vi "Check Refnum Class.vi"(8 "error in (no error)":errorcluster, 11 "Ring Field in":refnum<class "Ring Field.lvclass">) -> (0 "error out":errorcluster, 3 "Ring Field out":refnum<class "Ring Field.lvclass">)   [LabVIEW 2020, in "Basic Fields.lvlib" / "Ring Field.lvclass"]
uses:
  Ring Field.lvclass
  C:/Users/User/Desktop/Raman Program/Database OOP/source/Field/Field Class/Field.lvclass
  Field/Field Class/Field.lvclass/Field.ctl
  Field/Field Class/Field.lvclass
panel:
  # "For override: make sure that the wired control refnum class matches the field child class"
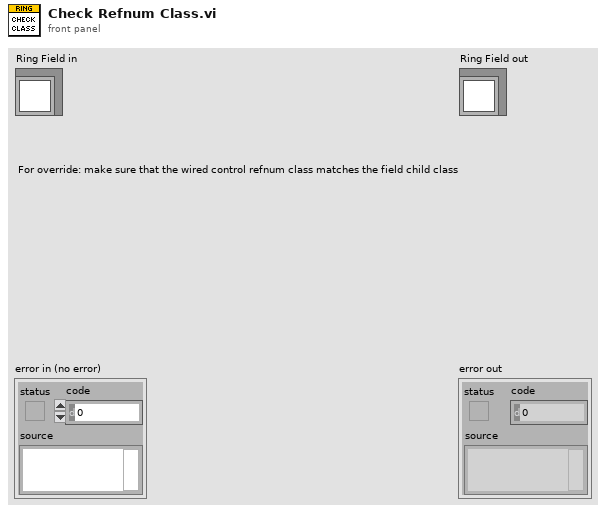
[diagram p1: front panel]
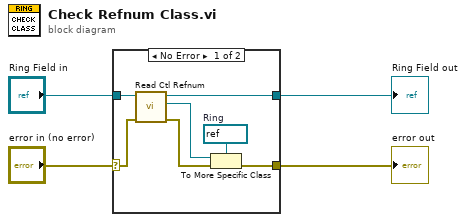
[diagram p0: block diagram]
diagram:
  n1 = case shown="No Error" "error in (no error)" {
    selector: "error in (no error)" -> [w9 w12]
    tunnel: "Ring Field in" -> [w11 w13]
    tunnel: [w10 w13] -> w2
    tunnel: [w5 w12] -> w1
    frame No Error {
      w6 = refnum<vi> refnum  # Ring
      n2 = call "Read Ctl Refnum.vi"("error in (no error)"=w9, "Field in"=w11) -> ("error out"=w8:errorcluster, "Ctl Refnum"=w7:refnum<vi>, "Field out"=w10:refnum<class "Ring Field.lvclass">)  [unwired: 7 in]
      n3 = To More Specific Class(target class=w6, reference=w7, error in=w8) -> (error out=w5:errorcluster)  [unwired: 1 out]
    }
    frame Error {
    }
  }
  "error out" <- w1
  "Ring Field out" <- w2
